vi "subFD_Design & Analysis.vi"() -> ()   [LabVIEW 2023]
uses:
  <vilib>/addons/Digital Filter Design/_Objects.llb/DFD Pole-Zero Plot.ctl
  <vilib>/addons/Digital Filter Design/_Objects.llb/DFD Filter Obj.ctl
  <vilib>/addons/Digital Filter Design/_Objects.llb/DFD Filter Coef.ctl
  <vilib>/addons/Digital Filter Design/_Objects.llb/DFD Filter Structure Type Selector.ctl
  <vilib>/addons/Digital Filter Design/_Objects.llb/dfd_Internal Quantization Settings.ctl
  <vilib>/addons/Digital Filter Design/_Objects.llb/dfd_Internal Quantization Srcs.ctl
  <vilib>/addons/Digital Filter Design/_Objects.llb/DFD Coef Norm Type.ctl
  <vilib>/addons/Digital Filter Design/_Objects.llb/DFD Filter Frequence Specification (Design).ctl
  <vilib>/addons/Digital Filter Design/_Objects.llb/DFD Filter Ripple Specification (Design).ctl
  <vilib>/Utility/error.llb/ErrWarn.ctl
  <vilib>/addons/Digital Filter Design/_Objects.llb/DFD Phase Setting.ctl
  Instance           1 31Saved   subFD_Design & Analysis .vi
  <vilib>/addons/Digital Filter Design/FilterLib.llb/DFD Load Filter from File.vi
  <vilib>/addons/Digital Filter Design/Analysis.llb/DFD Plot Freq Response (Linear-Spaced).vi
  <vilib>/addons/Digital Filter Design/NI_DigFilterLicensed.lvlib
panel:
  in  "filter in":T1={"mSRate_Fs"=1.0, "mSRate_Version"="2.0", "mSRate_Comments"="", "mSRate_OrgCoef"={"type"=enum."Undefined", "gain"=1.0, "coef a (k)"=[], "coef b (v)"=[]}, "mSRate_CurCoef"={"type"=enum."Undefined", "gain"=1.0, "coef a (k)"=[], "coef b (v)"=[]}, "mSRate_Quantized?"=FALSE, "mSRate_QCoef"={"type"=enum."Undefined", "gain"=1.0, "coef a (k)"=[], "coef b (v)"=[]}, "mSRate_QSettings"=[], "mSRate_Order"=0, "mSRate_Scaling"={"mSRate_ScaleByPowerOf2?"=FALSE, "mSRate_ScaleType"=enum."No Norm"}} {"mSRate_QSettings"."source" items=["Coef a/k"=0, "Coef b/v"=7, "Input"=1, "Output"=2, "Multiplicand"=3, "Product"=4, "Sum"=5, "Delay"=6, "Gain"=8]}
  out "Status":string="Click the Design button to apply the new specifications."
  out "error":T7=TRUE
  in  "Unwrap?":bool=TRUE
  in  "Magnitude in dB?":bool=TRUE
  out "Filter Order":i32=-1
  in  "Graph Selector":u16(ring) items=["Magnitude", "Phase", "Group Delay", "Pole-Zero Plot", "Impulse Response"]
  out "Graph Tab":T8(tab)
  out "Magnitude Response":cluster{"f0":dbl, "df":dbl, "values":dbl[]}[](graph)
  out "Phase Response":cluster{"f0":dbl, "df":dbl, "values":dbl[]}[](graph)
  out "Group Delay":cluster{"f0":dbl, "df":dbl, "values":dbl[]}[](graph)
  out "Z-Plane":T9
  out "Coefficients":dbl[](graph)
  out "Successful Design?":bool
  in  "ripple specs":T10={"passband"=0.0, "stopband"=0.0, "dB/linear? (T: dB)"=TRUE}
  in  "freq specs [Hz]":T11
  out "filter out":T1={"mSRate_Fs"=1.0, "mSRate_Version"="1.0", "mSRate_Comments"="", "mSRate_OrgCoef"={"type"=enum."Undefined", "gain"=1.0, "coef a (k)"=[], "coef b (v)"=[]}, "mSRate_CurCoef"={"type"=enum."Undefined", "gain"=1.0, "coef a (k)"=[], "coef b (v)"=[]}, "mSRate_Quantized?"=FALSE, "mSRate_QCoef"={"type"=enum."Undefined", "gain"=1.0, "coef a (k)"=[], "coef b (v)"=[]}, "mSRate_QSettings"=[], "mSRate_Order"=0, "mSRate_Scaling"={"mSRate_ScaleByPowerOf2?"=FALSE, "mSRate_ScaleType"=enum."No Norm"}} {"mSRate_QSettings"."source" items=["Coef a/k"=0, "Coef b/v"=7, "Input"=1, "Output"=2, "Multiplicand"=3, "Product"=4, "Sum"=5, "Delay"=6, "Gain"=8]}
  out "OK":bool
  in  "stop":bool
  in  "Get a filter":T12(tab)
  in  "Design Method":u16(ring)=6 items=["Butterworth", "Chebyshev", "Inverse Chebyshev", "Elliptic", "Kaiser Window", "Dolph-Chebyshev Window", "Equi-Ripple FIR"]
  in  "fstop 1":dbl=12800.0 format="%#_5p Hz"
  in  "fpass 2":dbl=20000.0 format="%#_5p Hz"
  out "Filter Type":u16(ring)
  in  "Filter Type 2":u16(ring) items=["Lowpass", "Highpass", "Bandpass", "Bandstop"]
  in  "fs [Hz]":dbl=48000.0 format="%#_5p Hz"
  in  "fstop 2":dbl=16800.0 format="%#_5p Hz"
  in  "fpass 1":dbl=9600.0 format="%#_5p Hz"
  in  "Design":bool
  in  "Ripple Specifications in dB?":bool=TRUE
  in  "Stopband Attenuation":dbl=80.0 format="%#_5g"
  in  "Passband ripple":dbl=0.1 format="%#_5g"
  in  "Load Filter from File":bool
  out "Gain":dbl
  out "Coefficients Report":string
  # "Design Result"
  # "Filter Specifications"
  # "Frequency Specifications"
  # "Ripple Specifications"
  # "Status"
  # "Design Method"
  # "fstop 1"
  # "fpass 2"
  # "fs"
  # "fstop 2"
  # "fpass 1"
  # "Stopband\nAttenuation"
  # "Passband\nRipple"
  # "Design Result"
  # "Filter Information"
  # "Gain"
  # "Filter Coefficients Report"
  # "Status"
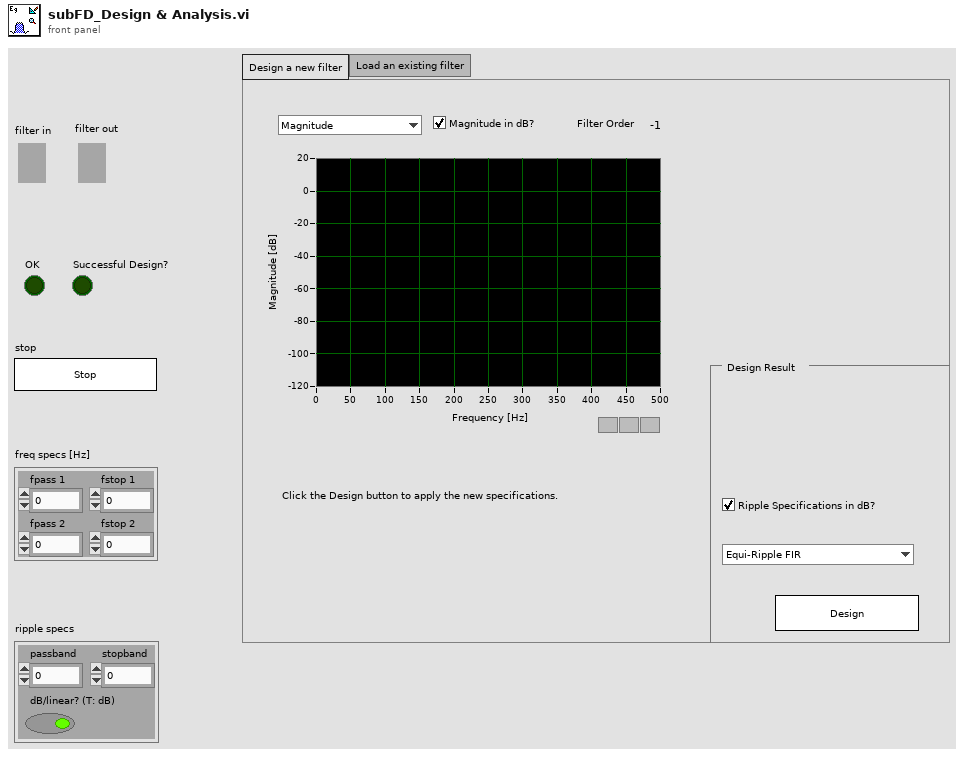
[diagram p1: front panel]
types:
  T1 = typedef "NI_DigFilterLicensed.lvlib/DFD Filter Obj.ctl" = cluster{"mSRate_Fs":dbl, "mSRate_Version":string, "mSRate_Comments":string, "mSRate_OrgCoef":T2, "mSRate_CurCoef":T2, "mSRate_Quantized?":bool, "mSRate_QCoef":T2, "mSRate_QSettings":T4[], "mSRate_Order":i32, "mSRate_Scaling":cluster{"mSRate_ScaleByPowerOf2?":bool, "mSRate_ScaleType":T6}}
  T2 = typedef "NI_DigFilterLicensed.lvlib/DFD Filter Coef.ctl" = cluster{"type":T3, "gain":dbl, "coef a (k)":dbl[], "coef b (v)":dbl[]}
  T3 = typedef "NI_DigFilterLicensed.lvlib/DFD Filter Structure Type Selector.ctl" = enum16{"Undefined", "FIR Direct Form", "FIR Direct Form Transposed", "FIR Symmetric", "FIR Antisymmetric", "IIR Direct Form I", "IIR Direct Form I Transposed", "IIR Direct Form II", "IIR Direct Form II Transposed", "IIR Cascaded Second Order Sections Form I", "IIR Cascaded Second Order Sections Form I Transposed", "IIR Cascaded Second Order Sections Form II", "IIR Cascaded Second Order Sections Form II Transposed", "Lattice Allpass (basic sections)", "Lattice Allpass (one multiplier sections)", "Lattice Allpass (normalized sections)", "Lattice AR (basic sections)", "Lattice AR (one multiplier sections)", "Lattice AR (normalized sections)", "Lattice MA (minimum phase)", "Lattice MA (maximum phase)", "Lattice ARMA (basic sections)", "Lattice ARMA (one multiplier sections)", "Lattice ARMA (normalized sections)"}
  T4 = typedef "NI_DigFilterLicensed.lvlib/dfd_Internal Quantization Settings.ctl" = cluster{"source":T5, "wl":i16, "iwl":i16, "overflow mode":enum16{"Saturation", "Wrap"}, "rounding mode":enum16{"Nearest", "Truncation"}, "signed?":bool}
  T5 = typedef "NI_DigFilterLicensed.lvlib/dfd_Internal Quantization Srcs.ctl" = u16
  T6 = typedef "NI_DigFilterLicensed.lvlib/DFD Coef Norm Type.ctl" = enum16{"No Norm", "Time Domain 1-Norm", "Time Domain 2-Norm", "Time Domain Inf-Norm"}
  T7 = typedef "ErrWarn.ctl" = bool
  T8 = enum32{"Magnitude", "Phase", "Group Delay", "Pole-Zero Plot", "Coefficients"}
  T9 = typedef "NI_DigFilterLicensed.lvlib/DFD Pole-Zero Plot.ctl" = cluster{dbl[], dbl[]}[]
  T10 = typedef "NI_DigFilterLicensed.lvlib/DFD Filter Ripple Specification (Design).ctl" = cluster{"passband":dbl, "stopband":dbl, "dB/linear? (T: dB)":bool}
  T11 = typedef "NI_DigFilterLicensed.lvlib/DFD Filter Frequence Specification (Design).ctl" = cluster{"fpass 1":dbl, "fstop 1":dbl, "fpass 2 ":dbl, "fstop 2":dbl}
  T12 = enum32{"Design a new filter", "Load an existing filter"}
  T13 = typedef "NI_DigFilterLicensed.lvlib/DFD Phase Setting.ctl" = cluster{"unwrap? (F)":bool, "degree? (F)":bool}
  T14 = cluster{"t0":dbl, "dt":dbl, "amplitudes":dbl[]}[]
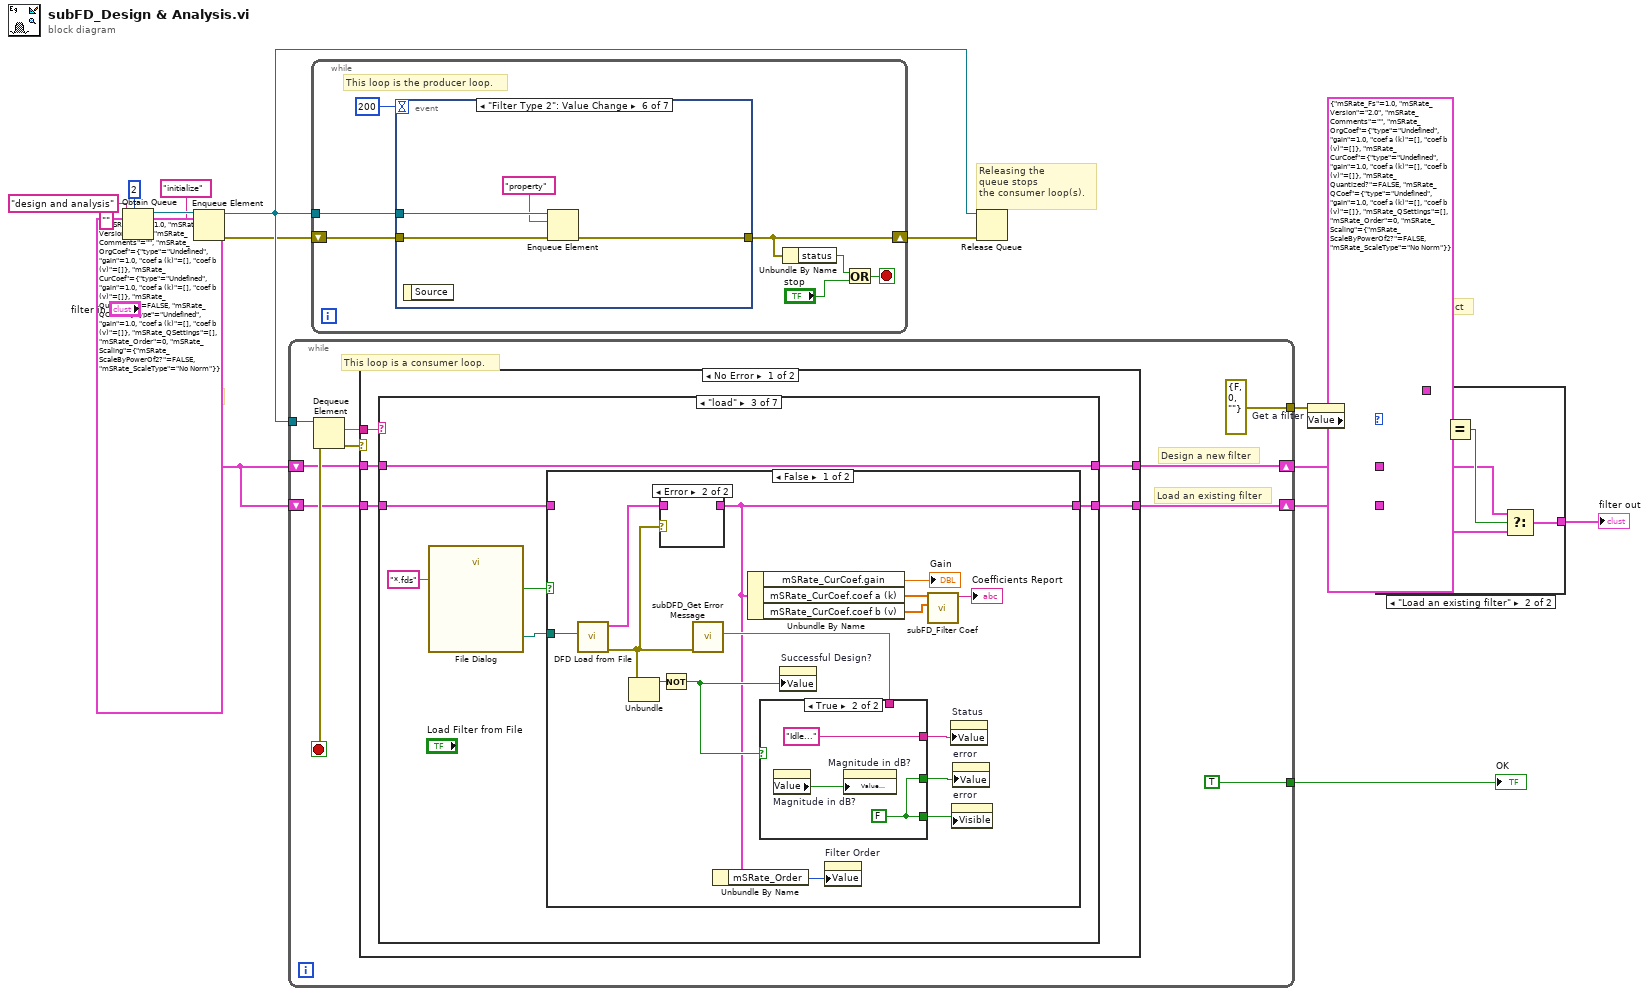
[diagram p0: block diagram]
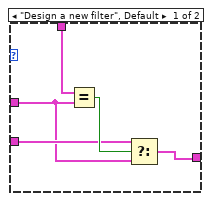
[diagram p2: hidden frame]
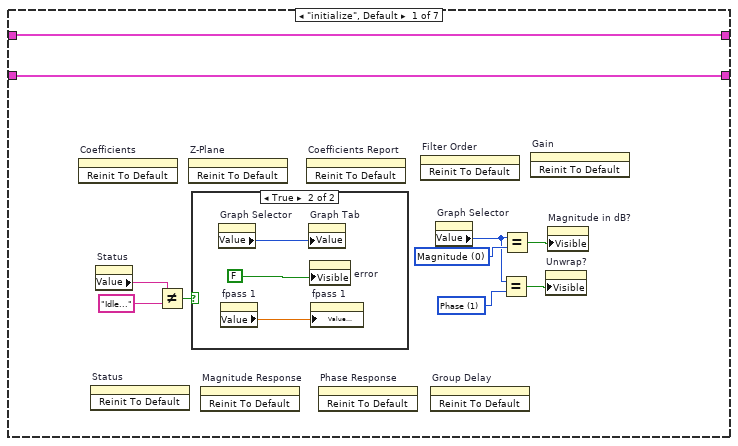
[diagram p3: hidden frame]
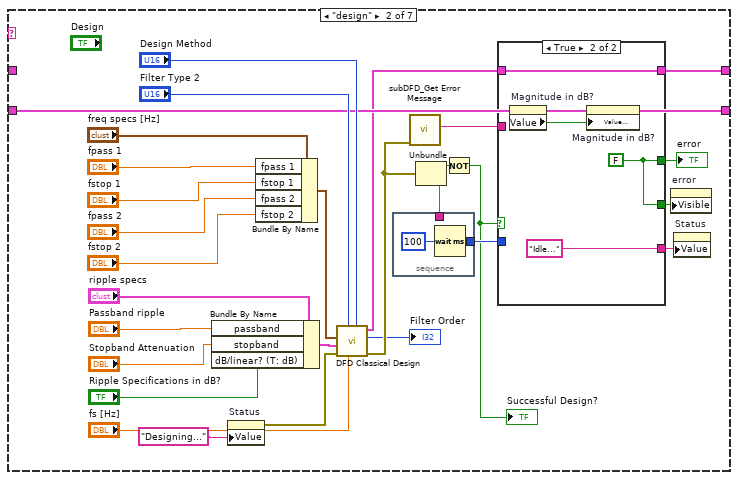
[diagram p5: hidden frame]
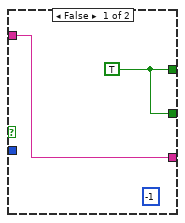
[diagram p6: hidden frame]
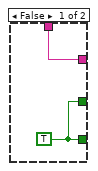
[diagram p8: hidden frame]
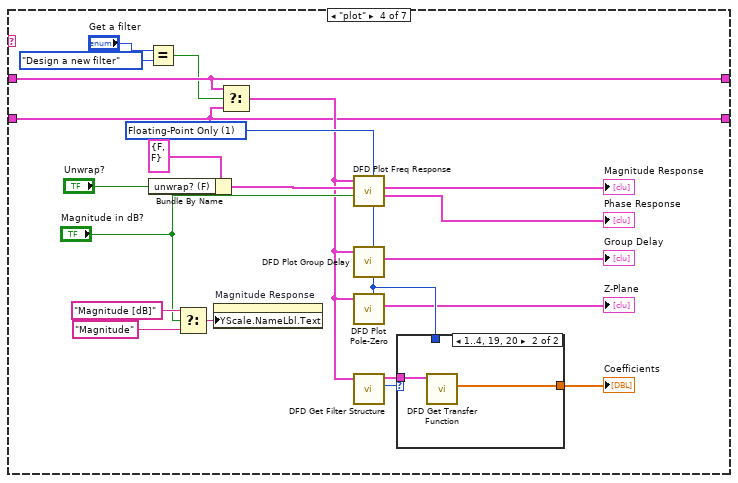
[diagram p10: hidden frame]
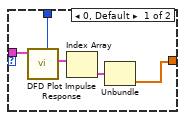
[diagram p11: hidden frame]
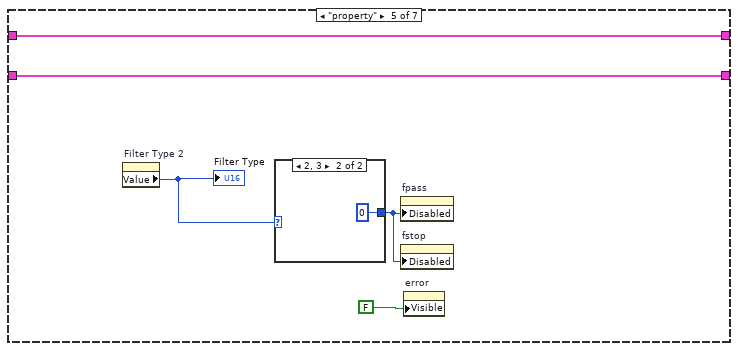
[diagram p12: hidden frame]
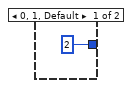
[diagram p13: hidden frame]
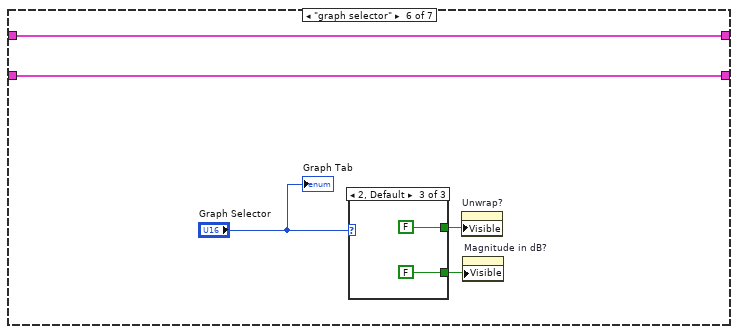
[diagram p14: hidden frame]
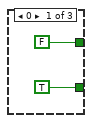
[diagram p15: hidden frame]
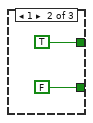
[diagram p16: hidden frame]
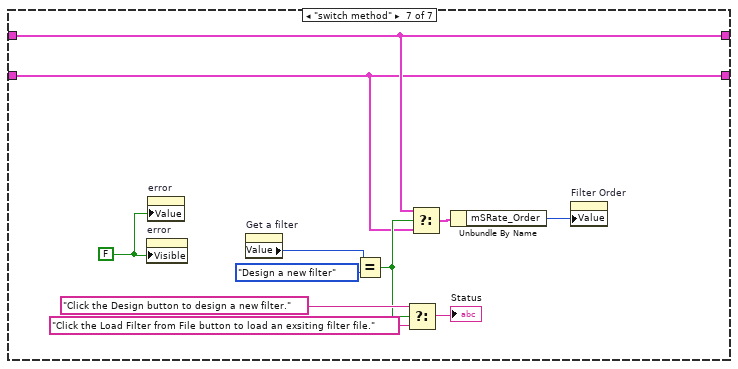
[diagram p17: hidden frame]
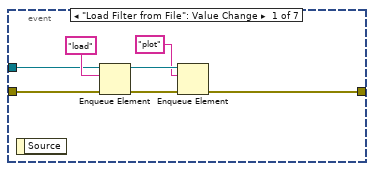
[diagram p19: hidden frame]
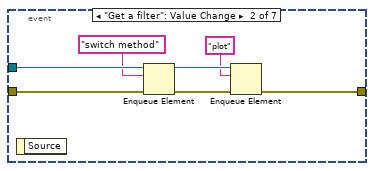
[diagram p20: hidden frame]
diagram:
  w8 = T1 {"mSRate_Fs"=1.0, "mSRate_Version"="2.0", "mSRate_Comments"="", "mSRate_OrgCoef"={"type"=enum."Undefined", "gain"=1.0, "coef a (k)"=[], "coef b (v)"=[]}, "mSRate_CurCoef"={"type"=enum."Undefined", "gain"=1.0, "coef a (k)"=[], "coef b (v)"=[]}, "mSRate_Quantized?"=FALSE, "mSRate_QCoef"={"type"=enum."Undefined", "gain"=1.0, "coef a (k)"=[], "coef b (v)"=[]}, "mSRate_QSettings"=[], "mSRate_Order"=0, "mSRate_Scaling"={"mSRate_ScaleByPowerOf2?"=FALSE, "mSRate_ScaleType"=enum."No Norm"}} ("filter out")
  # "empty filter object"
  # "empty filter object"
  # "Releasing the\nqueue stops\nthe consumer loop(s)."
  n1 = Obtain Queue(max queue size (-1, unlimited)=2, name (unnamed)="design and analysis", element data type="" ("name (unnamed)")) -> (queue out=w13:refnum<queue>, error out=w14:errorcluster)  [unwired: 2 in, 1 out]
  n2 = Enqueue Element(queue=w13, element="initialize", error in (no error)=w14) -> (queue out=w7:refnum<queue>, error out=w6:errorcluster)  [unwired: 2 out]
  n3 = while {
    tunnel: w7 -> [w26]
    shift-right: [w23] -> w4
    shift-left: w8 -> [w22]
    tunnel: [TRUE] -> w11
    shift-right: [w19] -> w3
    shift-left: w8 -> [w20]
    tunnel: [errorcluster {"status"=FALSE, "code"=0, "source"=""} ("error in (no error)")] -> w9
    stop <- w25 stop-if-true
    # "Load an existing filter"
    # "Design a new filter"
    # "This loop is a consumer loop."
    n4 = Dequeue Element(queue=w26) -> (element=w24:string, error out=w25:errorcluster)  [unwired: 1 in, 3 out]
    n5 = case shown="No Error" w25 {
      tunnel: w24 -> [w31 _]
      tunnel: [w30 w168] -> w23
      tunnel: w22 -> [w29 w168]
      tunnel: w20 -> [w28 w167]
      tunnel: [w27 w167] -> w19
      frame No Error {
        n6 = case shown="\"load\"" w31 {
          tunnel: [w33 w47 w84 w111 w139 w149 w159] -> w30
          tunnel: w29 -> [w33 _ w84 w111 w139 w149 w159]
          tunnel: w28 -> [w32 w51 w83 w112 w138 w145 w158]
          tunnel: [w32 w51 w82 w112 w138 w145 w158] -> w27
          frame "initialize", Default {
            w36 = u16 1 items=["Magnitude", "Phase", "Group Delay", "Pole-Zero Plot", "Impulse Response"] ("Graph Selector")
            w38 = u16 0 items=["Magnitude", "Phase", "Group Delay", "Pole-Zero Plot", "Impulse Response"] ("Graph Selector")
            n7 = invoke on="Coefficients" class="WFGraph (strict)" method="Reinit To Default"() -> ()  [unwired: 3 in, 3 out]
            n8 = invoke on="Status" class="Str" method="Reinit To Default"() -> ()  [unwired: 3 in, 3 out]
            n9 = property on="Status" class="Str"() -> ("Value"=w39:string)  [unwired: 2 in, 2 out]
            n10 = Not Equal?(x=w39, y="Idle...") -> (x != y?=w41:bool)
            n11 = invoke on="Z-Plane" class="XYGraph (strict)" method="Reinit To Default"() -> ()  [unwired: 3 in, 3 out]
            n12 = case shown="True" w41 {
              frame False {
              }
              frame True {
                n13 = property on="Graph Selector" class="Ring (strict)"() -> ("Value"=w43:u16)  [unwired: 2 in, 2 out]
                n14 = property on="fpass 1" class="DigNum (strict)"() -> ("Value"=w44:dbl)  [unwired: 2 in, 2 out]
                n15 = property on="Graph Tab" class="TabCtl (strict)"("Value"=w43) -> ()  [unwired: 2 in, 2 out]
                n16 = property on="error" class="Bool"("Visible"=FALSE) -> ()  [unwired: 2 in, 2 out]
                n17 = property on="fpass 1" class="DigNum (strict)"("Value (Signaling)"=w44) -> ()  [unwired: 2 in, 2 out]
              }
            }
            n18 = invoke on="Magnitude Response" class="WFGraph (strict)" method="Reinit To Default"() -> ()  [unwired: 3 in, 3 out]
            n19 = invoke on="Coefficients Report" class="Str" method="Reinit To Default"() -> ()  [unwired: 3 in, 3 out]
            n20 = invoke on="Phase Response" class="WFGraph (strict)" method="Reinit To Default"() -> ()  [unwired: 3 in, 3 out]
            n21 = invoke on="Filter Order" class="DigNum (strict)" method="Reinit To Default"() -> ()  [unwired: 3 in, 3 out]
            n22 = invoke on="Group Delay" class="WFGraph (strict)" method="Reinit To Default"() -> ()  [unwired: 3 in, 3 out]
            n23 = property on="Graph Selector" class="Ring (strict)"() -> ("Value"=w34:u16)  [unwired: 2 in, 2 out]
            n24 = Equal?(x=w34, y=w36) -> (x = y?=w35:bool)
            n25 = Equal?(x=w34, y=w38) -> (x = y?=w37:bool)
            n26 = invoke on="Gain" class="DigNum (strict)" method="Reinit To Default"() -> ()  [unwired: 3 in, 3 out]
            n27 = property on="Unwrap?" class="Bool (strict)"("Visible"=w35) -> ()  [unwired: 2 in, 2 out]
            n28 = property on="Magnitude in dB?" class="Bool (strict)"("Visible"=w37) -> ()  [unwired: 2 in, 2 out]
          }
          frame "design" {
            n29 = Bundle By Name(cluster="ripple specs", "passband"="Passband ripple", "stopband"="Stopband Attenuation", "dB/linear? (T: dB)"="Ripple Specifications in dB?") -> (w58:T10)
            n30 = property on="Status" class="Str"("Value"="Designing..." ("status")) -> (error out=w63:errorcluster)  [unwired: 2 in, 1 out]
            n31 = Bundle By Name(cluster="freq specs [Hz]", "fpass 1"="fpass 1", "fstop 1"="fstop 1", "fpass 2"="fpass 2", "fstop 2"="fstop 2") -> (w57:T11)
            n32 = call <vilib>:"DFD Classical Design.vi"("design method"="Design Method", "fs [Hz]"="fs [Hz]", "filter type"="Filter Type 2", "error in (no error)"=w63, "ripple specs"=w58, "freq specs [Hz]"=w57) -> ("error out"=w73:errorcluster, "order"=→"Filter Order":i32, "filter out"=w48:T1)  [unwired: 3 out]
            n33 = call <vilib>:"subDFD_Get Error Message.vi"("error in (no error)"=w73) -> ("Error Message"=w49:string)  [unwired: 10 out]
            n34 = Unbundle(w73) -> ("status"=w60:bool, "source"=w65:string)  [unwired: 1 out]
            n35 = stacked-sequence {
              tunnel: w65 -> [_]
              tunnel: [w74] -> w66
              frame #0 {
                n36 = Wait (ms)(milliseconds to wait=u32 100) -> (millisecond timer value=w74:u32)
              }
            }
            n37 = Not(x=w60) -> (.not. x?=w61:bool)
            "Successful Design?" <- w61
            n38 = case shown="True" w61 {
              tunnel: [w77 "Idle..." ("status")] -> w64
              tunnel: w66 -> [_ _]
              tunnel: w49 -> [w77 _]
              tunnel: w48 -> [_ w79]
              tunnel: [_ w79] -> w47
              tunnel: [w76 w78] -> w46
              tunnel: [w76 w78] -> w45
              frame False {
                (unwired) -1 ("order")
                w76 = T7 TRUE ("error")
              }
              frame True {
                w78 = T7 FALSE ("error")
                n39 = property on="Magnitude in dB?" class="Bool (strict)"() -> ("Value"=w81:bool)  [unwired: 2 in, 2 out]
                n40 = property on="Magnitude in dB?" class="Bool (strict)"("Value (Signaling)"=w81) -> ()  [unwired: 2 in, 2 out]
              }
            }
            "error" <- w46
            n41 = property on="error" class="Bool"("Visible"=w45) -> ()  [unwired: 2 in, 2 out]
            n42 = property on="Status" class="Str"("Value"=w64) -> ()  [unwired: 2 in, 2 out]
          }
          frame "load" {
            n43 = call "File Dialog"("pattern (all files)"="*.fds") -> ("selected path"=w87:path, "cancelled"=w86:bool)  [unwired: 6 in, 7 out]
            n44 = case shown="False" w86 {
              tunnel: w87 -> [w102 _]
              tunnel: w83 -> [_ w109]
              tunnel: [w91 w109] -> w82
              frame False {
                n45 = call-poly <vilib>:"DFD Load from File.vi"("file path in"=w102) -> ("error out"=w93:errorcluster, "filter out"=w92:T1)  [unwired: 1 in, 8 out]
                n46 = Unbundle(w93) -> ("status"=w101:bool)  [unwired: 2 out]
                n47 = case shown="Error" w93 {
                  tunnel: w92 -> [w103 _]
                  tunnel: [w103 _] -> w91
                  frame No Error {
                  }
                  frame Error {
                  }
                }
                n48 = Not(x=w101) -> (.not. x?=w100:bool)
                n49 = call <vilib>:"subDFD_Get Error Message.vi"("error in (no error)"=w93) -> ("Error Message"=w99:string)  [unwired: 10 out]
                n50 = Unbundle By Name(w91) -> ("mSRate_Order"=w90:i32)
                n51 = Unbundle By Name(w91) -> ("mSRate_CurCoef.gain"=→"Gain":dbl, "mSRate_CurCoef.coef a (k)"=w97:dbl[], "mSRate_CurCoef.coef b (v)"=w96:dbl[])
                n52 = case shown="True" w100 {
                  tunnel: [w105 "Idle..." ("status")] -> w94
                  tunnel: w99 -> [w105 _]
                  tunnel: [w104 w106] -> w89
                  tunnel: [w104 w106] -> w88
                  frame False {
                    w104 = TRUE ("Visible")
                  }
                  frame True {
                    w106 = FALSE ("Visible")
                    n53 = property on="Magnitude in dB?" class="Bool (strict)"() -> ("Value"=w108:bool)  [unwired: 2 in, 2 out]
                    n54 = property on="Magnitude in dB?" class="Bool (strict)"("Value (Signaling)"=w108) -> ()  [unwired: 2 in, 2 out]
                  }
                }
                n55 = property on="Successful Design?" class="Bool (strict)"("Value"=w100) -> ()  [unwired: 2 in, 2 out]
                n56 = property on="Filter Order" class="DigNum (strict)"("Value"=w90) -> ()  [unwired: 2 in, 2 out]
                n57 = call "subFD_Filter Coef.vi"("Coef b (v)"=w96, "Coef a (k)"=w97) -> ("Coefficients Report"=→"Coefficients Report":string)  [unwired: 9 out]
                n58 = property on="Status" class="Str"("Value"=w94) -> ()  [unwired: 2 in, 2 out]
                n59 = property on="error" class="Bool"("Visible"=w89) -> ()  [unwired: 2 in, 2 out]
                n60 = property on="error" class="Bool"("Value"=w88) -> ()  [unwired: 2 in, 2 out]
              }
              frame True {
              }
            }
          }
          frame "plot" {
            w126 = u16 1 items=["Auto", "Floating-Point Only", "Fixed-Point Only"] ("output option")
            n61 = Equal?(x="Get a filter", y=T12."Design a new filter") -> (x = y?=w110:bool)
            n62 = Bundle By Name(cluster=T13 {"unwrap? (F)"=FALSE, "degree? (F)"=FALSE} ("phase view"), "unwrap? (F)"="Unwrap?") -> (w119:T13)
            n63 = Select(t="Magnitude [dB]", s="Magnitude in dB?", f="Magnitude") -> (s? t:f=w129:string)
            n64 = property on="Magnitude Response" class="WFGraph (strict)"("YScale.NameLbl.Text"=w129) -> ()  [unwired: 2 in, 2 out]
            n65 = Select(t=w111, s=w110, f=w112) -> (s? t:f=w113:T1)
            n66 = call-poly <vilib>:"DFD Plot Freq Response.vi"("output option"=w126, "dB on? (T)"="Magnitude in dB?", "phase view"=w119, "filter in"=w113) -> ("phase response"=→"Phase Response":cluster{"f0":dbl, "df":dbl, "values":dbl[]}[], "magnitude response"=→"Magnitude Response":cluster{"f0":dbl, "df":dbl, "values":dbl[]}[])  [unwired: 4 in, 2 out]
            n67 = call <vilib>:"DFD Plot Group Delay.vi"("output option"=w126, "filter in"=w113) -> ("group delay"=→"Group Delay":cluster{"f0":dbl, "df":dbl, "values":dbl[]}[])  [unwired: 3 in, 6 out]
            n68 = call <vilib>:"DFD Plot Pole-Zero.vi"("output option"=w126, "filter in"=w113) -> ("Z-Plane"=→"Z-Plane":T9)  [unwired: 2 in, 7 out]
            n69 = call <vilib>:"DFD Get Filter Structure.vi"("filter in"=w113) -> ("structure"=w123:u16, "filter out"=w124:T1)  [unwired: 1 in, 8 out]
            n70 = case shown="1..4, 19, 20" w123 {
              tunnel: w124 -> [w135 w137]
              tunnel: [w132 w136] -> w125
              tunnel: w126 -> [w131 _]
              frame 0, Default {
                n71 = call <vilib>:"DFD Plot Impulse Response.vi"("output option"=w131, "filter in"=w135) -> ("impulse response"=w134:T14)  [unwired: 3 in, 6 out]
                n72 = Index Array(array=w134) -> (element=w133:cluster{"t0":dbl, "dt":dbl, "amplitudes":dbl[]})  [unwired: 1 in]
                n73 = Unbundle(w133) -> ("amplitudes"=w132:dbl[])  [unwired: 2 out]
              }
              frame 1..4, 19, 20 {
                n74 = call <vilib>:"DFD Get Transfer Function.vi"("filter in"=w137) -> ("numerator"=w136:dbl[])  [unwired: 1 in, 9 out]
              }
            }
            "Coefficients" <- w125
          }
          frame "property" {
            n75 = property on="Filter Type 2" class="Ring (strict)"() -> ("Value"=w140:u16)  [unwired: 2 in, 2 out]
            "Filter Type" <- w140
            n76 = case shown="2, 3" w140 {
              tunnel: [u8 2 ("Disabled") u8 0 ("Disabled")] -> w141
              frame 0, 1, Default {
              }
              frame 2, 3 {
              }
            }
            n77 = property on="fpass" class="DigNum (strict)"("Disabled"=w141) -> ()  [unwired: 2 in, 2 out]
            n78 = property on="fstop" class="DigNum (strict)"("Disabled"=w141) -> ()  [unwired: 2 in, 2 out]
            n79 = property on="error" class="Bool"("Visible"=FALSE) -> ()  [unwired: 2 in, 2 out]
          }
          frame "graph selector" {
            n80 = case shown="2, Default" "Graph Selector" {
              tunnel: [FALSE TRUE FALSE] -> w146
              tunnel: [TRUE FALSE FALSE] -> w147
              frame 0 {
              }
              frame 1 {
              }
              frame 2, Default {
              }
            }
            n81 = property on="Unwrap?" class="Bool (strict)"("Visible"=w146) -> ()  [unwired: 2 in, 2 out]
            n82 = property on="Magnitude in dB?" class="Bool (strict)"("Visible"=w147) -> ()  [unwired: 2 in, 2 out]
            "Graph Tab" <- "Graph Selector"
          }
          frame "switch method" {
            w160 = FALSE ("Visible")
            n83 = property on="error" class="Bool"("Visible"=w160) -> ()  [unwired: 2 in, 2 out]
            n84 = property on="error" class="Bool"("Value"=w160) -> ()  [unwired: 2 in, 2 out]
            n85 = property on="Get a filter" class="TabCtl (strict)"() -> ("Value"=w165:T12)  [unwired: 2 in, 2 out]
            n86 = Equal?(x=w165, y=T12."Design a new filter") -> (x = y?=w161:bool)
            n87 = Select(t="Click the Design button to design a new filter.", s=w161, f="Click the Load Filter from File button to load an exsiting filter file.") -> (s? t:f=→"Status":string)
            n88 = Select(t=w159, s=w161, f=w158) -> (s? t:f=w157:T1)
            n89 = Unbundle By Name(w157) -> ("mSRate_Order"=w156:i32)
            n90 = property on="Filter Order" class="DigNum (strict)"("Value"=w156) -> ()  [unwired: 2 in, 2 out]
          }
        }
      }
      frame Error {
      }
    }
  }
  "OK" <- w11
  n91 = while {
    shift-right: [w172] -> w17
    shift-left: w6 -> [w174]
    tunnel: w7 -> [w175]
    stop <- w173 stop-if-true
    # "This loop is the producer loop."
    n92 = event shown="[5] \"Filter Type 2\": Value Change" {
      selector: _ -> [_ _ _ _ _ _ _]
      dyn-events: _ -> [_ _ _ _ _ _ _]
      timeout: 200 -> [_ _ _ _ _ _ _]
      tunnel: w175 -> [w181 w188 w193 w196 w203 w207 _]
      tunnel: w174 -> [w180 w189 w192 w199 w202 w206 w208]
      tunnel: [w178 w185 w194 w198 w201 w205 w208] -> w172
      event "Load Filter from File": Value Change {
        n93 = event-data() -> ()  [unwired: 2 out]
        n94 = Enqueue Element(queue=w181, element="load", error in (no error)=w180) -> (queue out=w177:refnum<queue>, error out=w179:errorcluster)  [unwired: 2 out]
        n95 = Enqueue Element(queue=w177, element="plot", error in (no error)=w179) -> (error out=w178:errorcluster)  [unwired: 3 out]
      }
      event "Get a filter": Value Change {
        n96 = event-data() -> ()  [unwired: 2 out]
        n97 = Enqueue Element(queue=w188, element="switch method" ("f"), error in (no error)=w189) -> (queue out=w184:refnum<queue>, error out=w186:errorcluster)  [unwired: 2 out]
        n98 = Enqueue Element(queue=w184, element="plot" ("f"), error in (no error)=w186) -> (error out=w185:errorcluster)  [unwired: 3 out]
      }
      event "Design": Value Change {
        n99 = event-data() -> ()  [unwired: 2 out]
        n100 = Enqueue Element(queue=w193, element="design", error in (no error)=w192) -> (queue out=w191:refnum<queue>, error out=w194:errorcluster)  [unwired: 2 out]
        n101 = Enqueue Element(queue=w191, element="plot") -> ()  [unwired: 1 in, 4 out]
      }
      event "Unwrap?", "Magnitude in dB?": Value Change {
        n102 = event-data() -> ()  [unwired: 2 out]
        n103 = Enqueue Element(queue=w196, element="plot", error in (no error)=w199) -> (error out=w198:errorcluster)  [unwired: 3 out]
      }
      event "Graph Selector": Value Change {
        n104 = event-data() -> ()  [unwired: 2 out]
        n105 = Enqueue Element(queue=w203, element="graph selector", error in (no error)=w202) -> (error out=w201:errorcluster)  [unwired: 3 out]
      }
      event "Filter Type 2": Value Change {
        n106 = event-data() -> ()  [unwired: 2 out]
        n107 = Enqueue Element(queue=w207, element="property", error in (no error)=w206) -> (error out=w205:errorcluster)  [unwired: 3 out]
      }
      event Timeout {
        n108 = event-data() -> ()  [unwired: 2 out]
      }
    }
    n109 = Unbundle By Name(w172) -> ("status"=w171:bool)
    n110 = Or(x=w171, y="stop") -> (x .or. y?=w173:bool)
  }
  n111 = Release Queue(queue=w7, error in (no error)=w17) -> ()  [unwired: 4 out]
  n112 = property on="Get a filter" class="TabCtl (strict)"(error in=w9) -> ("Value"=w5:T12)  [unwired: 1 in, 2 out]
  n113 = case shown="\"Load an existing filter\"" w5 {
    tunnel: w4 -> [w210 w215]
    tunnel: w3 -> [w211 w216]
    tunnel: T1 {"mSRate_Fs"=1.0, "mSRate_Version"="2.0", "mSRate_Comments"="", "mSRate_OrgCoef"={"type"=enum."Undefined", "gain"=1.0, "coef a (k)"=[], "coef b (v)"=[]}, "mSRate_CurCoef"={"type"=enum."Undefined", "gain"=1.0, "coef a (k)"=[], "coef b (v)"=[]}, "mSRate_Quantized?"=FALSE, "mSRate_QCoef"={"type"=enum."Undefined", "gain"=1.0, "coef a (k)"=[], "coef b (v)"=[]}, "mSRate_QSettings"=[], "mSRate_Order"=0, "mSRate_Scaling"={"mSRate_ScaleByPowerOf2?"=FALSE, "mSRate_ScaleType"=enum."No Norm"}} ("filter out") -> [w213 w217]
    tunnel: [w209 w214] -> w1
    frame "Design a new filter", Default {
      n114 = Equal?(x=w213, y=w210) -> (x = y?=w212:bool)
      n115 = Select(t=w211, s=w212, f=w210) -> (s? t:f=w209:T1)
    }
    frame "Load an existing filter" {
      n116 = Equal?(x=w217, y=w216) -> (x = y?=w218:bool)
      n117 = Select(t=w215, s=w218, f=w216) -> (s? t:f=w214:T1)
    }
  }
  "filter out" <- w1
